vi "Continuous B sweep.vi"(6 "Mode":T5, 7 "Rate (T/min)":dbl=0.0125 min=0.0 max=0.2, 8 "error in (no error)":errorcluster, 9 "Simulate/Run":enum16{"simulate mode", "run mode"}(ring), 10 "Min (start)":dbl=1.0 min=-8.0 max=8.0, 11 "Max (end)":dbl=-1.0 min=-8.0 max=8.0) -> (0 "error out":errorcluster)   [LabVIEW 2019, in "Sweep Control.lvclass"]
uses:
  Sweep Control.lvclass
  Typedefs/Enum - Experiments.ctl
  Typedefs/Continuous B Sweep JSON--Cluster.ctl
  <userlib>/LevyLab/Instrument Framework/Instrument Types/Cryostat/Instrument.Cryostat.lvclass
  <userlib>/LevyLab/Transport/Transport/Transport.lvclass
  <userlib>/LevyLab/Transport/Control Experiment/Control Experiment.lvclass
  <userlib>/LevyLab/Lockin-Multichannel/Instrument.Lockin/Instrument.Lockin.lvclass
  <userlib>/LevyLab/Transport/Control Experiment/Typedefs/Instrument Classes--cluster.ctl
  <userlib>/LevyLab/Transport/Control Experiment/Typedefs/Wiring Description--cluster.ctl
  <userlib>/LevyLab/Transport/Control Experiment/Typedefs/Instrument--enum.ctl
  <userlib>/LevyLab/Transport/Control Experiment/Typedefs/Experiment Description--cluster.ctl
  <userlib>/LevyLab/Instrument Framework/Instrument Types/VSource/Instrument.VSource.lvclass
  <userlib>/LevyLab/Instrument Framework/Instrument Types/VNA/Instrument.VNA.lvclass
  <userlib>/LevyLab/Instrument Framework/Instrument Types/Strain/Instrument.Strain.lvclass
  <userlib>/LevyLab/Instrument Framework/Instrument Types/CBridge/Instrument.CBridge.lvclass
  <userlib>/LevyLab/Lockin-Multichannel/Instrument.DAQ/Typedefs/Sweep.Pattern--Enum.ctl
  <userlib>/LevyLab/Lockin-Multichannel/Instrument.DAQ/Instrument.DAQ.lvclass
  <userlib>/LevyLab/Lockin-Multichannel/Instrument.DAQ/Typedefs/Sweep.Channel--Cluster.ctl
  <userlib>/LevyLab/Instrument Framework/Instrument Types/Delay Line/Instrument.DelayLine.lvclass
  <userlib>/LevyLab/Transport/Control Experiment/Typedefs/Instrument Types--combo.ctl
  <userlib>/LevyLab/Lockin-Multichannel/Instrument.DAQ/Typedefs/REF.Channel--Cluster.ctl
  <userlib>/LevyLab/Lockin-Multichannel/Instrument.DAQ/Typedefs/REF.Channel--Cluster--Array.ctl
  <userlib>/LevyLab/Lockin-Multichannel/Instrument.DAQ/Typedefs/AO.Channel.Function--Enum.ctl
  <userlib>/LevyLab/Lockin-Multichannel/Instrument.DAQ/Typedefs/AO.Channel--Cluster.ctl
  <userlib>/LevyLab/Lockin-Multichannel/Instrument.DAQ/Typedefs/AO.Channel--Cluster--Array.ctl
  65c9b652-50f2-4ab4-8260-00ea008a43cc.vi
  <userlib>/LevyLab/Transport/Control Experiment/Typedefs/Instruments--cluster.ctl
  <userlib>/LevyLab/Krohn Hite 7008/SMOs/Inst.Krohn-Hite-7008/Inst.Krohn-Hite-7008.lvclass
  <userlib>/LevyLab/Krohn Hite 7008/SMOs/KH7008/typedefs/Filter--Enum.ctl
  <userlib>/LevyLab/Krohn Hite 7008/SMOs/KH7008/KH7008.lvlib
  <userlib>/LevyLab/Krohn Hite 7008/SMOs/KH7008/typedefs/couple--Enum.ctl
  <userlib>/LevyLab/Krohn Hite 7008/SMOs/KH7008/typedefs/shunt--enum.ctl
  <userlib>/LevyLab/Krohn Hite 7008/SMOs/KH7008/typedefs/Input--Enum.ctl
  <userlib>/LevyLab/Krohn Hite 7008/SMOs/KH7008/typedefs/gain--enum.ctl
  <userlib>/LevyLab/Krohn Hite 7008/SMOs/KH7008/typedefs/channel--numeric.ctl
  <userlib>/LevyLab/Krohn Hite 7008/SMOs/KH7008/typedefs/channelProperties--Cluster.ctl
  <userlib>/LevyLab/Krohn Hite 7008/SMOs/KH7008/typedefs/allChannelProperties--Array.ctl
  <userlib>/LevyLab/Instrument Framework/Instrument Types/Cryostat/Typedefs/Magnet Mode--Enum.ctl
  <userlib>/LevyLab/Lockin-Multichannel/Instrument.DAQ/Typedefs/Sweep.Channel--Cluster--Array.ctl
  <userlib>/LevyLab/Transport/Transport/Typedefs/Lockin_Sweep JSON--Cluster.ctl
panel:
  in  "Lockin_sweep Configuration":T1[](array[typedef]) {"Sweep Tables"."Table" format="%#_3p"; "Sweep Tables"."Ch" min=1 max=16; "Sweep Channels"."Table" format="%#_1f"; "Sweep Channels"."Channel" min=1 max=128; "Sweep Channels"."Start" format="%#_6p"; "Sweep Channels"."End" format="%#_6p"}
  out "Setpoint (T)":dbl=1.0
  in  "Experiment Folder":string="49-LockinFieldSweep"
  in  "Experiment subVI":T6
  in  "Experiment Description":string="Lockin measurements at different X and Y gate values\n\n- lockin channel 17,18,19,20: leads 3,8,15,27 (x,y,-x,-y gates)\ngate combinations:\nx2,y2,x1,y1\n0,0,0,0\n17.5,0,-17.5,0\n-17.5,0,17.5,0\n0,17.5,0,-17.5\n0,-17.5,0,17.5\n17.5,0,17.5,0\n0,17.5,0,17.5\n\n-Vbg = lead 26: 0V\n-T: 20mK\n-B=1T to -1T @0.0125T/min and vice versa\n\n400nm periodicity hash\n\nLockin channel 2,1: leads 5,4 , current mode, SR: 5kOhm, Gain:1000x\nLockin channel 2: lead 5: Vac:1mV, Vdc:0V, freq: 13Hz\nLockin channel 3,4: leads 6,7 , voltage mode SR: open, Gain:1000x\n\nsolid rectangle\n    \nLockin channel 5,8: leads 9,13 , current mode, SR: 5kOhm, Gain:1000x\nLockin channel 5: lead 9: Vac:1mV, Vdc:0V, freq: 13Hz\nLockin channel 6,7: leads 11,12 , voltage mode SR: open, Gain:1000x\n\n\n200nm periodicity hash\n\nLockin channel 12,11: leads 21,20 , current mode, SR: 5kOhm, Gain:1000x\nLockin channel 12: lead 21: Vac:1mV, Vdc:0V, freq: 13Hz\nLockin channel 9,10: leads 16,17 , voltage mode SR: open, Gain:1000x\n\nAdditional lockin settings:\nLine filter on\nDecimation Factor: 10\nFs: 65000\n#s: 5000"
  out "time (minutes)":dbl=40.0
  out "ETA":timestamp=timestamp(3698546516.7356124 s since 1904-01-01) caption="Timestamp" format="%<%m/%d/%Y %I:%M:%S %p>T"
  out "time (hours)":dbl=2.0
  out "Step #":i32=1
  in  "Function":enum16{"Ramp", "Triangle", "Sine"}(ring)
  in  "Phase":dbl
  in  "Cycles (1,2,...)":i32=1 min=1 step=1
  in  "step size":dbl=2.0 format="%.4f"
  out "B Field Graph":cluster{i32[], dbl[]}[](graph)=[{[0, 1], [-1.0, 1.0]}, {[1], [1.0]}]
  in  "stop":bool
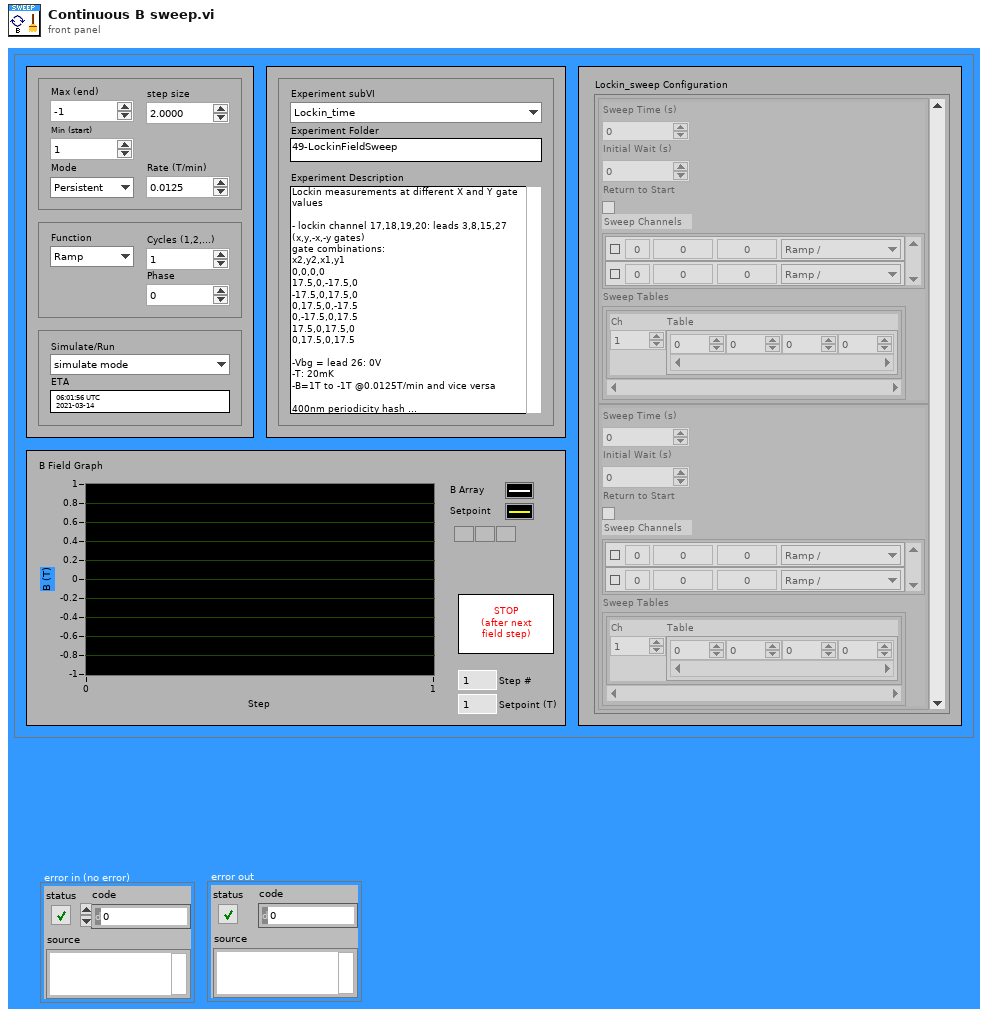
[diagram p1: front panel]
types:
  T1 = typedef "Transport.lvclass/Lockin_Sweep JSON--Cluster.ctl" = cluster{"Sweep Time (s)":dbl, "Initial Wait (s)":dbl, "Return to Start":bool, "Sweep Channels":T2, "Sweep Tables":cluster{"Ch":i32, "Table":dbl[]}[]}
  T2 = typedef "Instrument.DAQ.lvclass/Sweep.Channel--Cluster--Array.ctl" = T3[]
  T3 = typedef "Instrument.DAQ.lvclass/Sweep.Channel--Cluster.ctl" = cluster{"Enable?":bool, "Channel":u16, "Start":dbl, "End":dbl, "Pattern":T4, "Table":dbl[]}
  T4 = typedef "Instrument.DAQ.lvclass/Sweep.Pattern--Enum.ctl" = enum16{"Ramp /", "Ramp /\\", "Smooth Ramp _/", "Smooth Ramp _/\\_", "Table"}
  T5 = typedef "Instrument.Cryostat.lvclass/Magnet Mode--Enum.ctl" = enum16{"Persistent", "Driven"}
  T6 = typedef "Sweep Control.lvclass/Enum - Experiments.ctl" = enum16{"Lockin_time", "Lockin_sweep", "Lockin_DelayLine"}
  T7 = cluster{"Sweep Time (s)":dbl, "Initial Wait (s)":dbl, "Return to Start":bool, "Channels":T3[]}
  T8 = enum32{"Invalid", "Standard", "Closed", "Hidden", "Minimized", "Maximized"}
  T9 = enum32{"invalid app kind", "Development System", "Run Time System", "Student Edition", "Embedded LabVIEW", "Evaluation", "Custom"}
  T10 = typedef "Sweep Control.lvclass/Continuous B Sweep JSON--Cluster.ctl" = cluster{"Continuous B Sweep":cluster{"Experiment":T6, "B field values":dbl[]}, "Experiment Description":T11, "Wiring Configuration":T15, "Lockin":cluster{"AOconfig":T16, "REFconfig":T19}, "Krohn Hite":cluster{"Channel Setting":T21}}
  T11 = typedef "Control Experiment.lvclass/Experiment Description--cluster.ctl" = cluster{"User":string, "Device":string, "Device Path":path, "Device Description":string, "Experiment Path":path, "Experiment Description":string, "Instrument":T12, "Instruments":T13[], "Sweep":cluster{"key":string, "value":variant}[]}
  T12 = typedef "Control Experiment.lvclass/Instrument--enum.ctl" = enum16{"----- AFM/EBL -----", "AGILENT", "CYPHER", "Gemini2", "JEOL", "MFP3D", "----- Cryostat -----", "CF900", "DR200", "MNK", "PPMS (simulated)", "PPMS 1", "PPMS 2", "PPMS 3", "----- Optics -----", "THz 1 (Element 2/Montana)", "THz 2 (Tsunami/Janis)"}
  T13 = typedef "Control Experiment.lvclass/Instruments--cluster.ctl" = cluster{"class path":path, "Address":string, "Type":T14}
  T14 = typedef "Control Experiment.lvclass/Instrument Types--combo.ctl" = string
  T15 = typedef "Control Experiment.lvclass/Wiring Description--cluster.ctl" = cluster{"Lockin Ch":i32[], "KH":cluster{"Electrodes":string[], "Labels":string[]}, "not KH":cluster{"Electrodes":string[], "Labels":string[]}}
  T16 = typedef "Instrument.DAQ.lvclass/AO.Channel--Cluster--Array.ctl" = T17[]
  T17 = typedef "Instrument.DAQ.lvclass/AO.Channel--Cluster.ctl" = cluster{"Enable?":bool, "Channel":i32, "Amplitude":dbl, "Offset":dbl, "Frequency":dbl, "Phase":dbl, "Function":T18, "Sweeping?":bool}
  T18 = typedef "Instrument.DAQ.lvclass/AO.Channel.Function--Enum.ctl" = enum16{"Sine", "Triangle", "Square"}
  T19 = typedef "Instrument.DAQ.lvclass/REF.Channel--Cluster--Array.ctl" = T20[]
  T20 = typedef "Instrument.DAQ.lvclass/REF.Channel--Cluster.ctl" = cluster{"Enable?":bool, "Channel":i32, "Frequency":dbl, "Phase":dbl, "TC":dbl, "Roll-Off":i32}
  T21 = typedef "KH7008.lvlib/allChannelProperties--Array.ctl" = T22[]
  T22 = typedef "KH7008.lvlib/channelProperties--Cluster.ctl" = cluster{"channel":T23, "gain":T24, "input":T25, "shunt":T26, "couple":T27, "filter":T28}
  T23 = typedef "KH7008.lvlib/channel--numeric.ctl" = u16
  T24 = typedef "KH7008.lvlib/gain--enum.ctl" = enum16{"1x", "10x", "100x", "1000x"}
  T25 = typedef "KH7008.lvlib/Input--Enum.ctl" = enum16{"OFF", "SE+", "SE-", "DIFF"}
  T26 = typedef "KH7008.lvlib/shunt--enum.ctl" = enum16{"Open", "50", "500", "5k", "50k", "10M"}
  T27 = typedef "KH7008.lvlib/couple--Enum.ctl" = enum16{"AC", "DC"}
  T28 = typedef "KH7008.lvlib/Filter--Enum.ctl" = enum16{"OFF", "ON"}
  T29 = typedef "Control Experiment.lvclass/Instrument Classes--cluster.ctl" = cluster{"KH7008":refnum<class "Inst.Krohn-Hite-7008.lvclass">, "Lockin":refnum<class "Instrument.Lockin.lvclass">, "Temperature":refnum<class "Instrument.Cryostat.lvclass">, "Magnet":refnum<class "Instrument.Cryostat.lvclass">, "Rotator":refnum<class "Instrument.Cryostat.lvclass">, "Level":refnum<class "Instrument.Cryostat.lvclass">, "Capacitance Bridge":refnum<class "Instrument.CBridge.lvclass">, "Delay Line":refnum<class "Instrument.DelayLine.lvclass">, "Strain Cell":refnum<class "Instrument.Strain.lvclass">, "VNA":refnum<class "Instrument.VNA.lvclass">, "Voltage Source":refnum<class "Instrument.VSource.lvclass">}
  T30 = cluster{"Core":cluster{"Current VI Reference":refnum<vi>, "Close Panel on Exit?":bool}, "SweepControl":refnum<class "Sweep Control.lvclass">, "ContinuousB_JSON":T10, "B field values":dbl[], "Sweep rate (T/min)":dbl, "Transport":refnum<class "Transport.lvclass">, "Instruments":T29, "Notifier":refnum<notifier>}
  T31 = cluster{"Current VI Reference":refnum<vi>, "Close Panel on Exit?":bool}
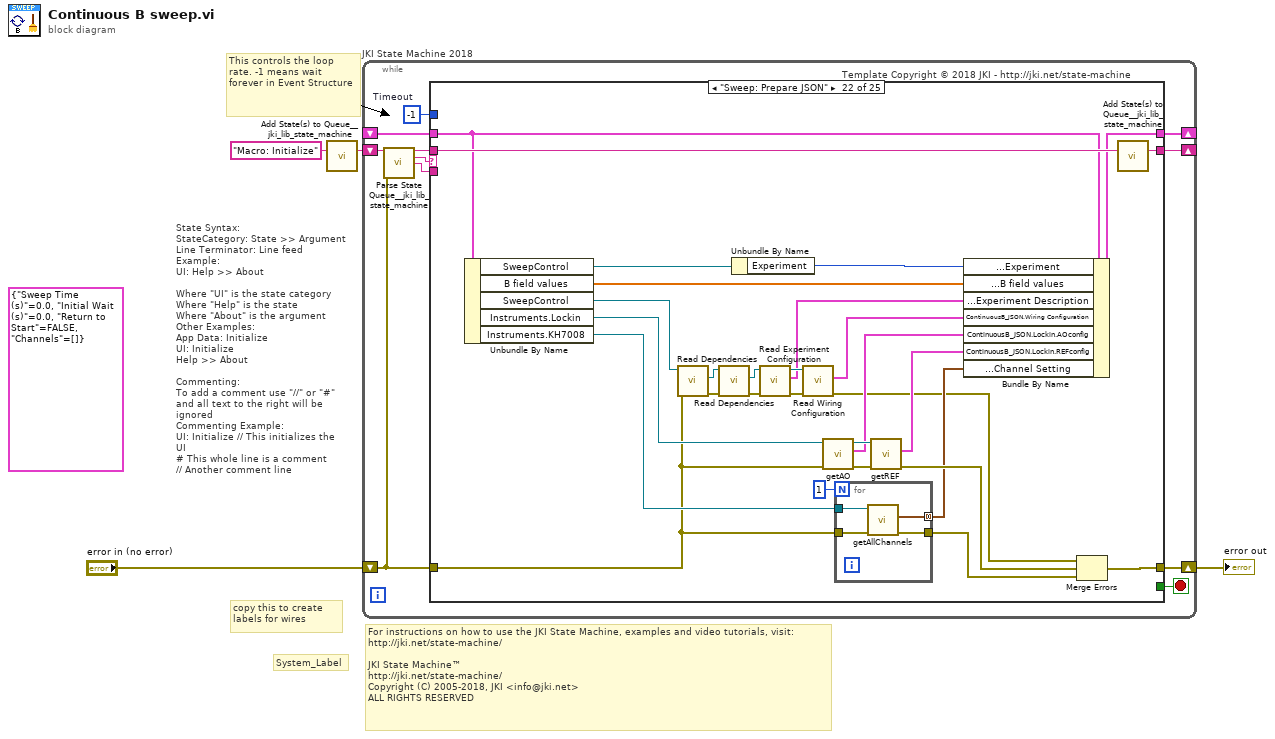
[diagram p0: block diagram]
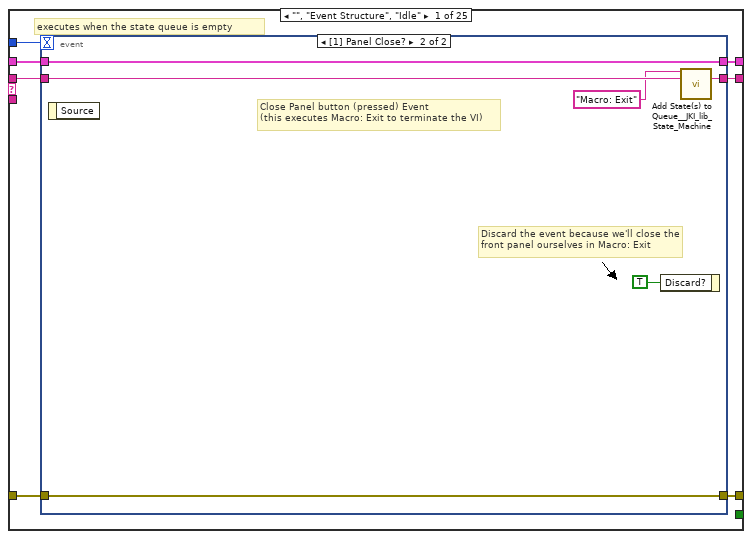
[diagram p2: hidden frame]
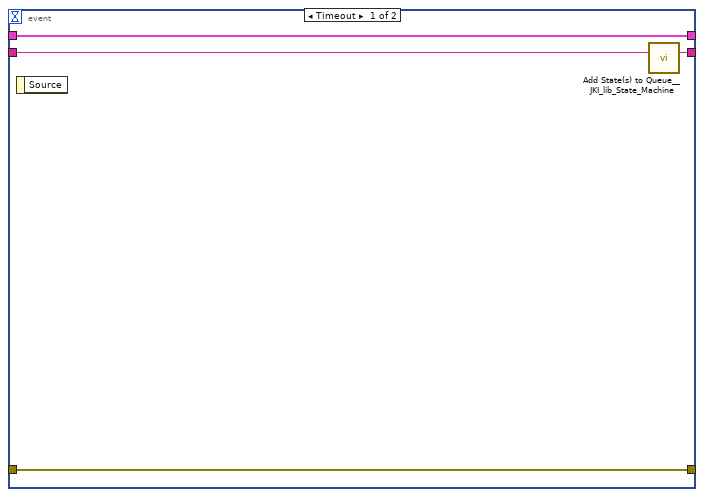
[diagram p3: hidden frame]
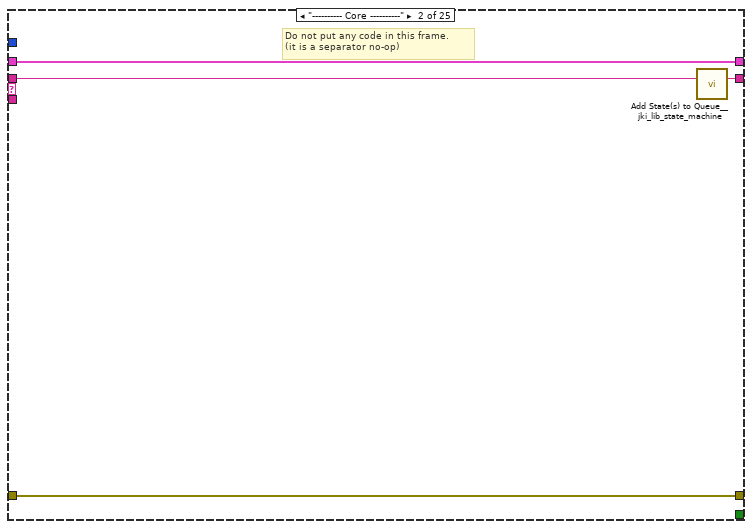
[diagram p4: hidden frame]
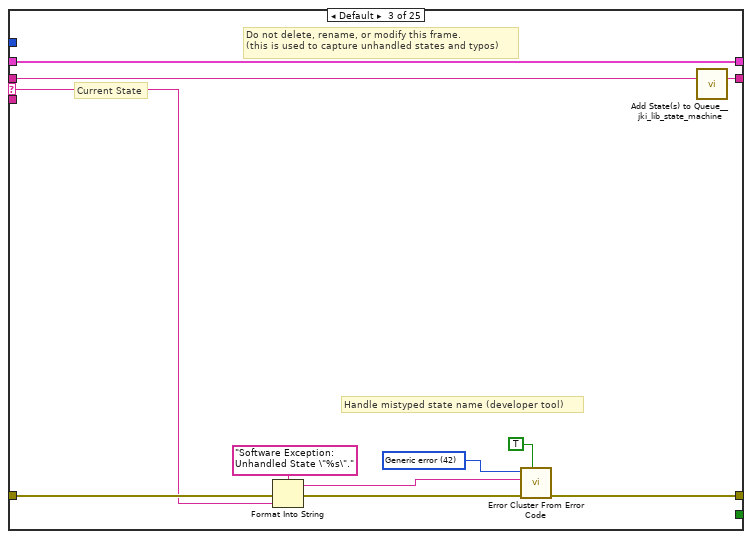
[diagram p5: hidden frame]
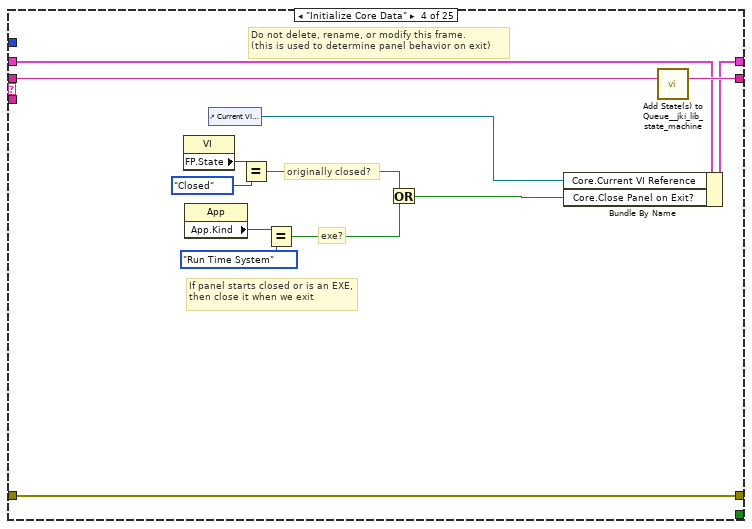
[diagram p6: hidden frame]
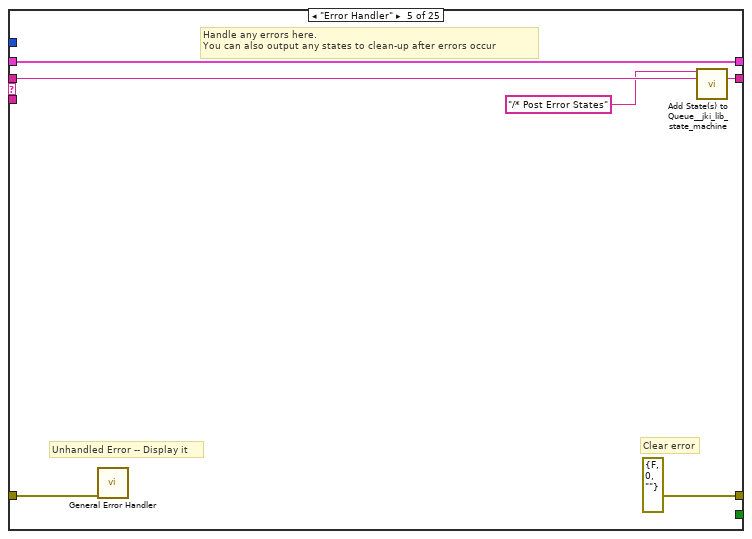
[diagram p7: hidden frame]
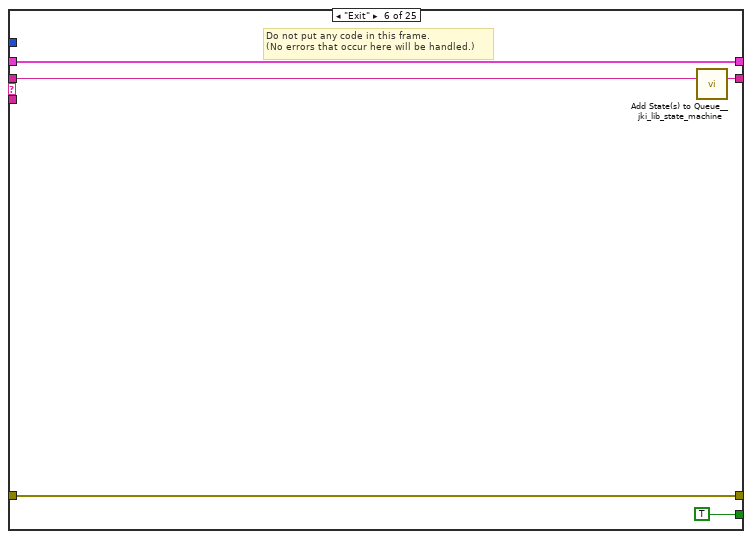
[diagram p8: hidden frame]
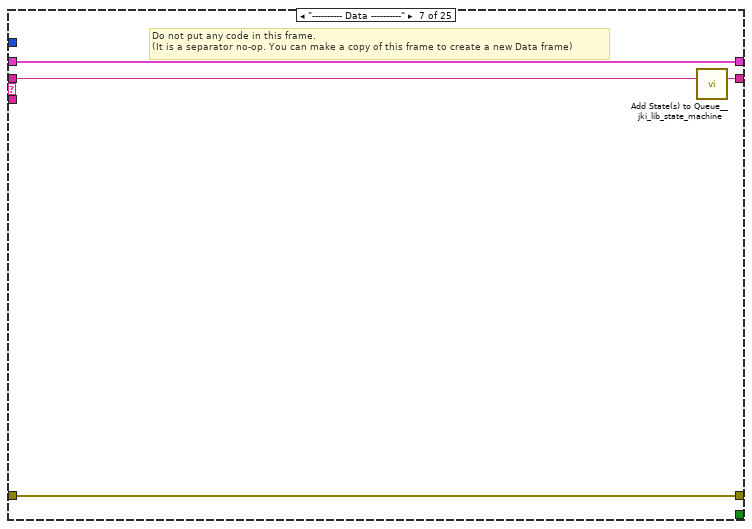
[diagram p9: hidden frame]
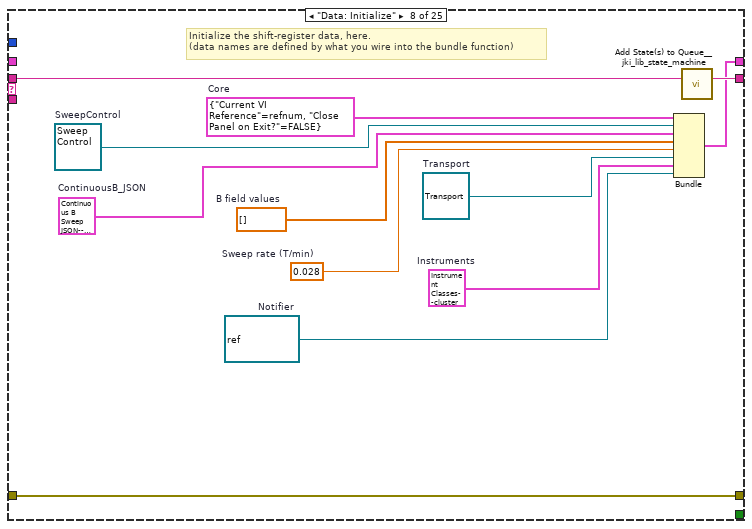
[diagram p10: hidden frame]
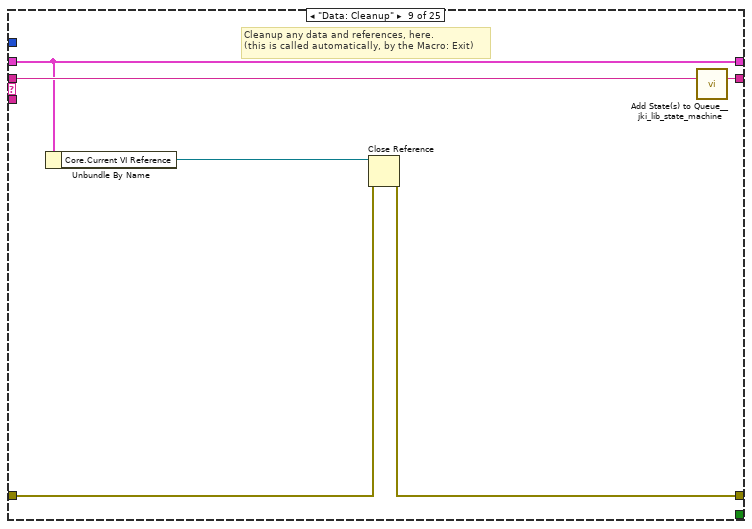
[diagram p11: hidden frame]
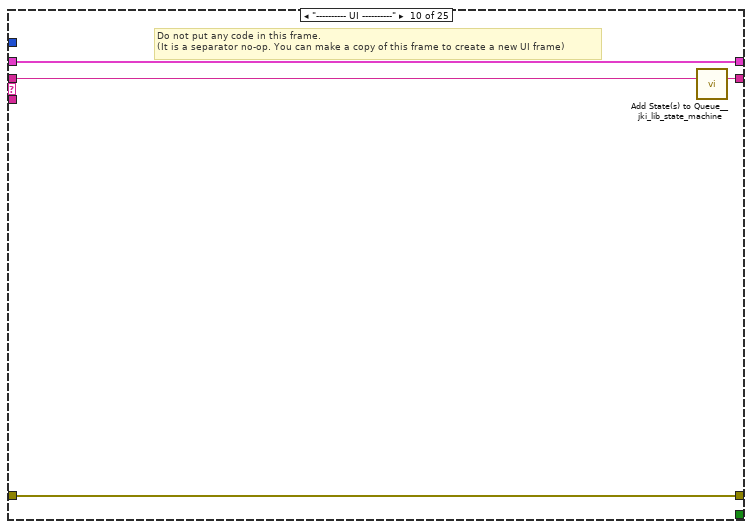
[diagram p12: hidden frame]
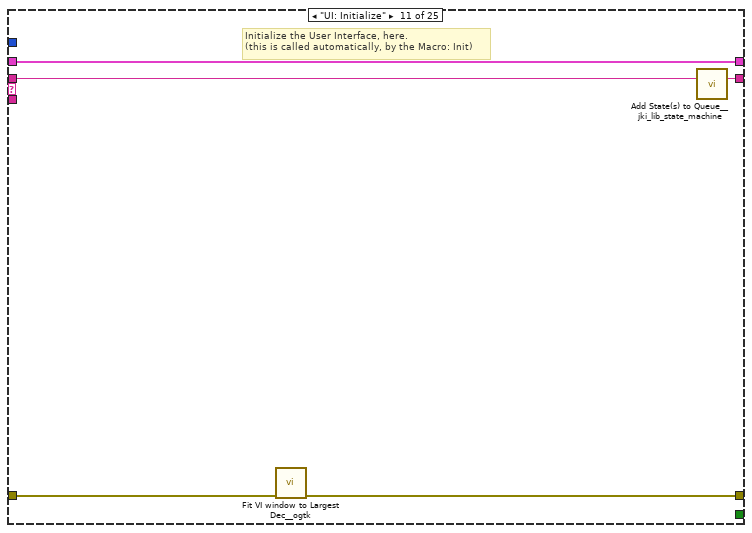
[diagram p13: hidden frame]
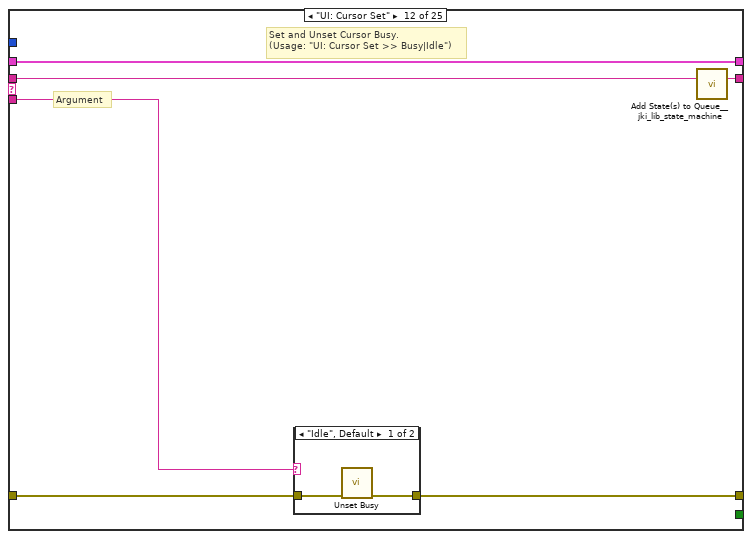
[diagram p14: hidden frame]
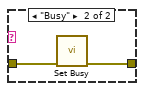
[diagram p15: hidden frame]
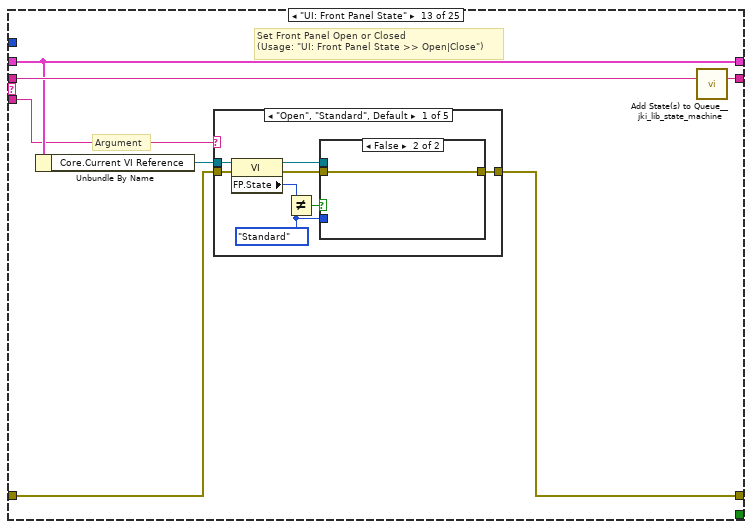
[diagram p16: hidden frame]
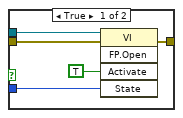
[diagram p17: hidden frame]
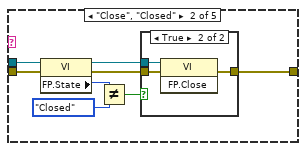
[diagram p18: hidden frame]
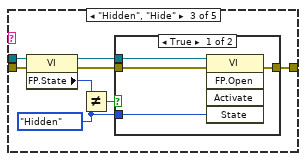
[diagram p20: hidden frame]
diagram:
  (unwired) T7 {"Sweep Time (s)"=0.0, "Initial Wait (s)"=0.0, "Return to Start"=FALSE, "Channels"=[]} ("Sweep")
  # "For instructions on how to use the JKI State Machine, examples and video tutorials, visit:\nhttp://jki.net/state-machine/\n\nJKI State Machine™\nhttp://jki.net/state-machine/\nCopyright (C) 2005-2018, JKI <info@jki.net>\nALL RIGHTS RESERVED"
  # "State Syntax:\nStateCategory: State >> Argument\nLine Terminator: Line feed\nExample:\nUI: Help >> About\n\nWhere \"UI\" is the state category\nWhere \"Help\" is the state\nWhere \"About\" is the argument\nOther Examples:\nApp Data: Initialize\nUI: Initialize\nHelp >> About\n\nCommenting:\nTo add a comment use \"//\" or \"#\" and all text to the right will be ignored\nCommenting Example:\nUI: Initialize // This initializes the UI\n# This whole line is a comment\n// Another comment line"
  # "copy this to create labels for wires"
  # "This controls the loop rate. -1 means wait forever in Event Structure"
  # "System_Label"
  n1 = call <vilib>:"Add State(s) to Queue__jki_lib_state_machine.vi"("State(s) in (\"\")"="Macro: Initialize") -> ("States Out"=w4:string)  [unwired: 14 in]
  n2 = while "JKI State Machine 2018" {
    shift-right: [w8] -> _
    shift-left: _ -> [w7]
    shift-right: [w11] -> w1
    shift-left: "error in (no error)" -> [w5]
    shift-right: [w10] -> _
    shift-left: w4 -> [w12]
    stop <- w9 stop-if-true
    w6 = -1  # Timeout
    # "Template Copyright © 2018 JKI - http://jki.net/state-machine"
    n3 = call <vilib>:"Parse State Queue__jki_lib_state_machine.vi"("State Queue"=w12, "Error In (no error)"=w5) -> ("Remaining States"=w14:string, "Current State"=w15:string, "Arguments"=w13:string)  [unwired: 11 in]
    n4 = case shown="\"Sweep: Prepare JSON\"" w15 {
      selector: w15 -> [_ _ w37 _ _ _ _ _ _ _ _ _ _ _ _ _ _ _ _ _ _ _ _ _ _]
      tunnel: w14 -> [w22 w36 w41 w60 w66 w71 w75 w87 w93 w97 w102 w108 w119 w188 w193 w199 w211 w215 w234 w260 w274 w303 w331 w348 w387]
      tunnel: w13 -> [_ _ _ _ _ _ _ _ _ _ _ w103 w113 _ _ _ _ _ _ _ _ _ _ _ _]
      tunnel: w7 -> [w20 w33 w39 w53 w63 w69 w72 _ w88 w94 w100 w106 w115 w185 w190 w196 w208 w212 w224 w246 w270 w295 w329 w335 w372]
      tunnel: [w19 w34 w43 w57 errorcluster {"status"=FALSE, "code"=0, "source"=""} ("error out") w68 w73 w84 w89 w95 w98 w104 w116 w186 w191 w197 w209 w213 w222 w237 w268 w288 w313 w346 w377] -> w11
      tunnel: w5 -> [w18 w34 w42 w57 w62 w68 w73 w84 w90 w95 w99 w105 w117 w186 w191 w197 w209 w213 w222 w250 w269 w276 w318 w346 w380]
      tunnel: [w21 w35 w40 w59 w65 w70 w74 w86 w92 w96 w101 w107 w118 w187 w192 w198 w210 w214 w233 w259 w273 w302 w330 w347 w386] -> w10
      tunnel: [_ _ _ _ _ TRUE _ _ _ _ _ _ _ _ _ _ _ _ _ _ _ _ _ _ _] -> w9
      tunnel: [w17 w33 w39 w58 w63 w69 w72 w85 w88 w94 w100 w106 w115 w185 w190 w196 w208 w212 w232 w245 w271 w294 w328 w335 w371] -> w8
      tunnel: w6 -> [w16 _ _ _ _ _ _ _ _ _ _ _ _ _ _ _ _ _ _ _ _ _ _ _ _]
      frame "", "Event Structure", "Idle" {
        # "executes when the state queue is empty"
        n5 = event shown="[1] Panel Close?" {
          selector: _ -> [_ _]
          dyn-events: _ -> [_ _]
          timeout: w16 -> [_ _]
          tunnel: w22 -> [w26 w32]
          tunnel: [w25 w31] -> w21
          tunnel: w20 -> [w23 w29]
          tunnel: [w24 w30] -> w19
          tunnel: w18 -> [w24 w30]
          tunnel: [w23 w29] -> w17
          event Timeout {
            n6 = event-data() -> ()  [unwired: 1 in, 1 out]
            n7 = call <vilib>:"Add State(s) to Queue__JKI_lib_State_Machine.vi"("State(s) in (\"\")"=w26) -> ("States Out"=w25:string)  [unwired: 14 in]
          }
          event Panel Close? {
            # "Discard the event because we'll close the front panel ourselves in Macro: Exit"
            # "Close Panel button (pressed) Event\n(this executes Macro: Exit to terminate the VI)"
            n8 = event-data() -> ()  [unwired: 1 in, 1 out]
            n9 = event-data("Discard?"=TRUE) -> ()  [unwired: 1 in, 1 out]
            n10 = call <vilib>:"Add State(s) to Queue__JKI_lib_State_Machine.vi"("State(s) in Front (\"\")"="Macro: Exit", "State(s) in (\"\")"=w32) -> ("States Out"=w31:string)  [unwired: 13 in]
          }
        }
      }
      frame "---------- Core ----------" {
        # "Do not put any code in this frame.\n(it is a separator no-op)"
        n11 = call <vilib>:"Add State(s) to Queue__jki_lib_state_machine.vi"("State(s) in (\"\")"=w36) -> ("States Out"=w35:string)  [unwired: 14 in]
      }
      frame Default {
        w46 = 42 items=["No error", "Argument error", "Memory is full", "Out of zone", "End of file", "File already open", "Generic file I/O error", "File not found", "File permission error", "Disk is full", "Duplicate path", "Too many files open", "System feature not enabled", "Resource file not found", "Cannot add resource", "Resource not found", "Image not found", "Image memory error", "Pen does not exist", "Config type invalid", "Config token not found", "Config parse error", "Config memory error", "Bad external code format", "Bad external code offset", "External code not present", "Null window", "Destroy window error", "Null menu", "Print aborted", "Bad print record", "Print driver error", "Windows error during printing", "Memory error during printing", "Print dialog error", "Generic print error", "Invalid device refnum", "Device not found", "Device parameter error", "Device unit error", "Cannot open device", "Device call aborted", "Generic error", "Cancelled by user", "Object ID too low", "Object ID too high", "Object not in heap", "Unknown heap", "Unknown object (invalid DefProc)", "Unknown object (DefProc not in table)", "Message out of range", "Invalid (null) method", "Unknown message", "Manager call not supported", "Bad address", "Network operation in progress", "Network operation timed out", "Connection is busy", "Network attribute not supported", "Network error", "Address in use", "System out of memory", "Connection aborted", "Connection refused", "Not connected", "Already connected", "Connection closed", "Initialization error (interapplication manager)", "Bad occurrence", "Wait on unbound occurrence handler", "Occurrence queue overflow", "Datalog type conflict", "Unused", "Unrecognized type (interapplication manager)", "Memory corrupt", "Failed to make temporary DLL", "Old CIN version", "Drag socket not found", "Failed to load drop-object", "Failed to register OLE object", "Failed to release OLE object", "Format specifier type mismatch", "Unknown format specifier", "Too few format specifiers", "Too many format specifiers", "Scan failed", "Newer CIN version", "Error converting to variant", "Runtime menu error", "Password tampered", "Variant attribute not found", "Incompatible variant data type", "Event data is not available", "Event Store is not present", "Occurrence is not found", "Event Queue is not created", "Event info is not available", "Refnum passed is NULL", "Error retrieving Class GUID", "Error retrieving CoClass GUID", "Error retrieving TypeLib GUID.", "Bad built application magic bytes.", "Specific driver is different from the specific driver associated with the Logical Name.", "There is no session opened to the class driver.", "Max Error", "MAX - Error with config objects", "MAX - Error loading configuration", "MAX - Group not supported"]
        # "Current State"
        # "Do not delete, rename, or modify this frame.\n(this is used to capture unhandled states and typos)"
        # "Handle mistyped state name (developer tool)"
        n12 = Format Into String(format string="Software Exception: Unhandled State \"%s\"." ("message"), error in=w42, w37) -> (resulting string=w45:string, error out=w44:errorcluster)  [unwired: 1 in]
        n13 = call <vilib>:"Error Cluster From Error Code.vi"("show call chain? (False)"=TRUE, "error in (no error)"=w44, "error message (\"\")"=w45, "error code (0)"=w46) -> ("error out"=w43:errorcluster)  [unwired: 5 in]
        n14 = call <vilib>:"Add State(s) to Queue__jki_lib_state_machine.vi"("State(s) in (\"\")"=w41) -> ("States Out"=w40:string)  [unwired: 14 in]
      }
      frame "Initialize Core Data" {
        # "Do not delete, rename, or modify this frame.\n(this is used to determine panel behavior on exit)"
        # "originally closed?"
        # "exe?"
        # "If panel starts closed or is an EXE, then close it when we exit"
        n15 = property class="VI"() -> ("FP.State"=w50:T8)  [unwired: 2 in, 2 out]
        n16 = property class="App"() -> ("App.Kind"=w56:T9)  [unwired: 2 in, 2 out]
        n17 = control-ref of="Current VI Reference"() -> (w51:refnum<vi>)
        n18 = Equal?(x=w50, y=T8."Closed" ("Front Panel Window:State")) -> (x = y?=w48:bool)
        n19 = Equal?(x=w56, y=T9."Run Time System" ("Application:Kind")) -> (x = y?=w54:bool)
        n20 = Or(x=w48, y=w54) -> (x .or. y?=w52:bool)
        n21 = Bundle By Name(cluster=w53, "Core.Current VI Reference"=w51, "Core.Close Panel on Exit?"=w52) -> (w58:T30)
        n22 = call <vilib>:"Add State(s) to Queue__jki_lib_state_machine.vi"("State(s) in (\"\")"=w60) -> ("States Out"=w59:string)  [unwired: 14 in]
      }
      frame "Error Handler" {
        # "Unhandled Error -- Display it"
        # "Handle any errors here.\nYou can also output any states to clean-up after errors occur"
        # "Clear error"
        n23 = call <vilib>:"General Error Handler.vi"("error in (no error)"=w62) -> ()  [unwired: 10 in, 5 out]
        n24 = call <vilib>:"Add State(s) to Queue__jki_lib_state_machine.vi"("State(s) in Front (\"\")"="/* Post Error States", "State(s) in (\"\")"=w66) -> ("States Out"=w65:string)  [unwired: 13 in]
      }
      frame "Exit" {
        # "Do not put any code in this frame.\n(No errors that occur here will be handled.)"
        n25 = call <vilib>:"Add State(s) to Queue__jki_lib_state_machine.vi"("State(s) in (\"\")"=w71) -> ("States Out"=w70:string)  [unwired: 14 in]
      }
      frame "---------- Data ----------" {
        # "Do not put any code in this frame.\n(It is a separator no-op. You can make a copy of this frame to create a new Data frame)"
        n26 = call <vilib>:"Add State(s) to Queue__jki_lib_state_machine.vi"("State(s) in (\"\")"=w75) -> ("States Out"=w74:string)  [unwired: 14 in]
      }
      frame "Data: Initialize" {
        w76 = T10 {"Continuous B Sweep"={"Experiment"=enum."Lockin_DelayLine", "B field values"=[]}, "Experiment Description"={"User"="", "Device"="", "Device Path"=path "", "Device Description"="", "Experiment Path"=path "", "Experiment Description"="", "Instrument"=enum."PPMS 1", "Instruments"=[], "Sweep"=[]}, "Wiring Configuration"={"Lockin Ch"=[], "KH"={"Electrodes"=[], "Labels"=[]}, "not KH"={"Electrodes"=[], "Labels"=[]}}, "Lockin"={"AOconfig"=[], "REFconfig"=[]}, "Krohn Hite"={"Channel Setting"=[]}}  # ContinuousB_JSON
        w77 = T29 {"KH7008"=refnum, "Lockin"=refnum, "Temperature"=refnum, "Magnet"=refnum, "Rotator"=refnum, "Level"=refnum, "Capacitance Bridge"=refnum, "Delay Line"=refnum, "Strain Cell"=refnum, "VNA"=refnum, "Voltage Source"=refnum}  # Instruments
        w79 = refnum<class "Transport.lvclass"> refnum  # Transport
        w80 = refnum<class "Sweep Control.lvclass"> refnum  # SweepControl
        w78 = refnum<notifier> refnum  # Notifier
        w81 = 0.028  # Sweep rate (T/min)
        w82 = dbl[] []  # B field values
        w83 = T31 {"Current VI Reference"=refnum, "Close Panel on Exit?"=FALSE}  # Core
        # "Initialize the shift-register data, here.\n(data names are defined by what you wire into the bundle function)"
        n27 = Bundle("Core"=w83, "SweepControl"=w80, "ContinuousB_JSON"=w76, "B field values"=w82, "Sweep rate (T/min)"=w81, "Transport"=w79, "Instruments"=w77, "Notifier"=w78) -> (w85:T30)  [unwired: 1 in]
        n28 = call <vilib>:"Add State(s) to Queue__jki_lib_state_machine.vi"("State(s) in (\"\")"=w87) -> ("States Out"=w86:string)  [unwired: 14 in]
      }
      frame "Data: Cleanup" {
        # "Cleanup any data and references, here.\n(this is called automatically, by the Macro: Exit)"
        n29 = Unbundle By Name(w88) -> ("Core.Current VI Reference"=w91:refnum<vi>)
        n30 = Close Reference(reference=w91, error in (no error)=w90) -> (error out=w89:errorcluster)
        n31 = call <vilib>:"Add State(s) to Queue__jki_lib_state_machine.vi"("State(s) in (\"\")"=w93) -> ("States Out"=w92:string)  [unwired: 14 in]
      }
      frame "---------- UI ----------" {
        # "Do not put any code in this frame.\n(It is a separator no-op. You can make a copy of this frame to create a new UI frame)"
        n32 = call <vilib>:"Add State(s) to Queue__jki_lib_state_machine.vi"("State(s) in (\"\")"=w97) -> ("States Out"=w96:string)  [unwired: 14 in]
      }
      frame "UI: Initialize" {
        # "Initialize the User Interface, here.\n(this is called automatically, by the Macro: Init)"
        n33 = call <userlib>:"Fit VI window to Largest Dec__ogtk.vi"("error in (no error)"=w99) -> ("error out"=w98:errorcluster)  [unwired: 5 in, 1 out]
        n34 = call <vilib>:"Add State(s) to Queue__jki_lib_state_machine.vi"("State(s) in (\"\")"=w102) -> ("States Out"=w101:string)  [unwired: 14 in]
      }
      frame "UI: Cursor Set" {
        # "Argument"
        # "Set and Unset Cursor Busy.\n(Usage: \"UI: Cursor Set >> Busy|Idle\")"
        n35 = case shown="\"Idle\", Default" w103 {
          tunnel: w105 -> [w110 w112]
          tunnel: [w109 w111] -> w104
          frame "Idle", Default {
            n36 = call <vilib>:"Unset Busy.vi"("error in (no error)"=w110) -> ("error out"=w109:errorcluster)  [unwired: 10 in]
          }
          frame "Busy" {
            n37 = call <vilib>:"Set Busy.vi"("error in (no error)"=w112) -> ("error out"=w111:errorcluster)  [unwired: 9 in, 1 out]
          }
        }
        n38 = call <vilib>:"Add State(s) to Queue__jki_lib_state_machine.vi"("State(s) in (\"\")"=w108) -> ("States Out"=w107:string)  [unwired: 14 in]
      }
      frame "UI: Front Panel State" {
        # "Argument"
        # "Set Front Panel Open or Closed\n(Usage: \"UI: Front Panel State >> Open|Close\")"
        n39 = Unbundle By Name(w115) -> ("Core.Current VI Reference"=w114:refnum<vi>)
        n40 = case shown="\"Open\", \"Standard\", Default" w113 {
          tunnel: w117 -> [w125 w140 w151 w164 w177]
          tunnel: [w127 w141 w153 w166 w179] -> w116
          tunnel: w114 -> [w126 w138 w152 w165 w178]
          frame "Open", "Standard", Default {
            w120 = T8."Standard" ("State")
            n41 = property class="VI"(reference=w126, error in=w125) -> (reference out=w123:refnum<vi>, error out=w124:errorcluster, "FP.State"=w122:T8)
            n42 = Not Equal?(x=w122, y=w120) -> (x != y?=w121:bool)
            n43 = case shown="False" w121 {
              tunnel: [w131 w133] -> w127
              tunnel: w124 -> [w130 w133]
              tunnel: w123 -> [w129 _]
              tunnel: w120 -> [w128 _]
              frame True {
                n44 = invoke class="VI" method="FP.Open"(reference=w129, error in=w130, "Activate"=TRUE, "State"=w128) -> (error out=w131:errorcluster)  [unwired: 1 in, 4 out]
              }
              frame False {
              }
            }
          }
          frame "Close", "Closed" {
            n45 = property class="VI"(reference=w138, error in=w140) -> (reference out=w137:refnum<vi>, error out=w139:errorcluster, "FP.State"=w135:T8)
            n46 = Not Equal?(x=w135, y=T8."Closed" ("Front Panel Window:State")) -> (x != y?=w134:bool)
            n47 = case shown="True" w134 {
              tunnel: [w142 w145] -> w141
              tunnel: w139 -> [w142 w144]
              tunnel: w137 -> [_ w143]
              frame False {
              }
              frame True {
                n48 = invoke class="VI" method="FP.Close"(reference=w143, error in=w144) -> (error out=w145:errorcluster)  [unwired: 1 in, 2 out]
              }
            }
          }
          frame "Hidden", "Hide" {
            w146 = T8."Hidden" ("State")
            n49 = property class="VI"(reference=w152, error in=w151) -> (reference out=w149:refnum<vi>, error out=w150:errorcluster, "FP.State"=w148:T8)
            n50 = Not Equal?(x=w148, y=w146) -> (x != y?=w147:bool)
            n51 = case shown="True" w147 {
              tunnel: [w157 w158] -> w153
              tunnel: w150 -> [w156 w158]
              tunnel: w149 -> [w155 _]
              tunnel: w146 -> [w154 _]
              frame True {
                n52 = invoke class="VI" method="FP.Open"(reference=w155, error in=w156, "State"=w154) -> (error out=w157:errorcluster)  [unwired: 2 in, 4 out]
              }
              frame False {
              }
            }
          }
          frame "Minimize", "Minimized" {
            w159 = T8."Minimized" ("State")
            n53 = property class="VI"(reference=w165, error in=w164) -> (reference out=w162:refnum<vi>, error out=w163:errorcluster, "FP.State"=w161:T8)
            n54 = Not Equal?(x=w161, y=w159) -> (x != y?=w160:bool)
            n55 = case shown="True" w160 {
              tunnel: [w170 w171] -> w166
              tunnel: w163 -> [w169 w171]
              tunnel: w162 -> [w168 _]
              tunnel: w159 -> [w167 _]
              frame True {
                n56 = invoke class="VI" method="FP.Open"(reference=w168, error in=w169, "State"=w167) -> (error out=w170:errorcluster)  [unwired: 2 in, 4 out]
              }
              frame False {
              }
            }
          }
          frame "Maximize", "Maximized" {
            w172 = T8."Maximized" ("State")
            n57 = property class="VI"(reference=w178, error in=w177) -> (reference out=w175:refnum<vi>, error out=w176:errorcluster, "FP.State"=w174:T8)
            n58 = Not Equal?(x=w174, y=w172) -> (x != y?=w173:bool)
            n59 = case shown="True" w173 {
              tunnel: [w183 w184] -> w179
              tunnel: w176 -> [w182 w184]
              tunnel: w175 -> [w181 _]
              tunnel: w172 -> [w180 _]
              frame True {
                n60 = invoke class="VI" method="FP.Open"(reference=w181, error in=w182, "State"=w180) -> (error out=w183:errorcluster)  [unwired: 2 in, 4 out]
              }
              frame False {
              }
            }
          }
        }
        n61 = call <vilib>:"Add State(s) to Queue__jki_lib_state_machine.vi"("State(s) in (\"\")"=w119) -> ("States Out"=w118:string)  [unwired: 14 in]
      }
      frame "---------- Macro ----------" {
        # "Do not put any code in this frame.\n(It is a separator no-op. You can make a copy of this frame to create a new Macro frame)"
        n62 = call <vilib>:"Add State(s) to Queue__jki_lib_state_machine.vi"("State(s) in (\"\")"=w188) -> ("States Out"=w187:string)  [unwired: 14 in]
      }
      frame "Macro: Initialize" {
        w189 = "Data: Initialize\nInitialize Core Data\nUI: Initialize\nUI: Front Panel State >> Open\nMacro: Sweep"  # Data: Initialize Initialize Core Data UI: Initialize UI: Front Panel State >> Open Macro: Sweep
        # "Initialization Macro\n(This is called once, when the VI starts)"
        n63 = call <vilib>:"Add State(s) to Queue__jki_lib_state_machine.vi"("State(s) in Front (\"\")"=w189, "State(s) in (\"\")"=w193) -> ("States Out"=w192:string)  [unwired: 13 in]
      }
      frame "Macro: Sweep" {
        # "Do not put any code in this frame.\n(It is a separator no-op. You can make a copy of this frame to create a new Macro frame)"
        n64 = case shown="\"simulate mode\", Default" "Simulate/Run" {
          tunnel: ["Sweep: Initialize\nSweep: Simulate Sweep\nMacro: Exit" "Sweep: Initialize\nSweep: Initialize Sweep Control\nSweep: Initialize Transport\nSweep: Prepare JSON\nSweep: Write JSON\nSweep: Sweep\nMacro: Exit"] -> w195
          frame "simulate mode", Default {
          }
          frame "run mode" {
          }
        }
        n65 = call <vilib>:"Add State(s) to Queue__jki_lib_state_machine.vi"("State(s) in Front (\"\")"=w195, "State(s) in (\"\")"=w199) -> ("States Out"=w198:string)  [unwired: 13 in]
      }
      frame "Macro: Exit" {
        # "Exit Macro\n(This is called once, when the VI exits)"
        n66 = Unbundle By Name(w208) -> ("Core.Close Panel on Exit?"=w207:bool)
        n67 = Select(t="UI: Front Panel State >> Close", s=w207, f="") -> (s? t:f=w204:string)
        n68 = call <vilib>:"Add State(s) to Queue__JKI_lib_State_Machine.vi"("State(s) in (\"\")"=w204, "State(s) at Back (\"\")"="Data: Cleanup\nExit") -> ("States Out"=w202:string)  [unwired: 13 in]
        n69 = call <vilib>:"Add State(s) to Queue__jki_lib_state_machine.vi"("State(s) in Front (\"\")"=w202, "State(s) in (\"\")"=w211) -> ("States Out"=w210:string)  [unwired: 13 in]
      }
      frame "---------- Sweep ----------" {
        # "Template Separator\n(You can make a copy of, or modify, this frame)"
        n70 = call <vilib>:"Add State(s) to Queue__jki_lib_state_machine.vi"("State(s) in (\"\")"=w215) -> ("States Out"=w214:string)  [unwired: 14 in]
      }
      frame "Sweep: Initialize" {
        # "Your code here.\n(You can make a copy of, or modify, this frame)"
        n71 = call <userlib>:"Max_Min_conversion.vi"("Min"="Min (start)", "Max"="Max (end)") -> ("offset"=w227:dbl, "Amplitude"=w226:dbl)  [unwired: 8 in]
        n72 = call <userlib>:"Ramp.vi"("phase"="Phase", "function (ramp)"="Function", "cycles (1,2,...)"="Cycles (1,2,...)", "step size"="step size", "offset"=w227, "amplitude"=w226) -> ("Waveform Graph"=w220:dbl[])  [unwired: 3 in, 2 out]
        n73 = for {
          tunnel: w220 -> [w235] mode=indexing
          tunnel: [w236] -> w219 mode=indexing
          tunnel: [w235] -> w218 mode=indexing
          i -> [w236]
        }
        n74 = Bundle(w219, w218) -> (w217:cluster{i32[], dbl[]})  [unwired: 1 in]
        n75 = Build Array(w217) -> (→"B Field Graph":cluster{i32[], dbl[]}[])
        n76 = Bundle By Name(cluster=w224, "B field values"=w220, "Sweep rate (T/min)"="Rate (T/min)") -> (w232:T30)
        n77 = call <vilib>:"Add State(s) to Queue__jki_lib_state_machine.vi"("State(s) in (\"\")"=w234) -> ("States Out"=w233:string)  [unwired: 14 in]
      }
      frame "Sweep: Initialize Sweep Control" {
        # "Template Separator\n(You can make a copy of, or modify, this frame)"
        n78 = Unbundle By Name(w246) -> ("SweepControl"=w251:refnum<class "Sweep Control.lvclass">)
        n79 = call <userlib>:"Control Experiment FGV.vi"("Function"=enum16{"read", "write"}."read", "error in (no error)"=w250) -> ("error out"=w247:errorcluster, "Control Experiment.lvclass out"=w256:refnum<class "Control Experiment.lvclass">)  [unwired: 8 in]
        n80 = Bundle By Name(cluster=w251, "Experiment"="Experiment subVI") -> (w240:refnum<class "Sweep Control.lvclass">)
        n81 = call <userlib>:"Write Experiment Description.vi"("error in (no error)"=w247, "Experiment Description"="Experiment Description", "Control Experiment in"=w256) -> ("error out"=w248:errorcluster, "Control Experiment out"=w255:refnum<class "Control Experiment.lvclass">)  [unwired: 7 in]
        n82 = call <userlib>:"Write Experiment Folder.vi"("error in (no error)"=w248, "Experiment Folder"="Experiment Folder", "Control Experiment in"=w255) -> ("error out"=w249:errorcluster, "Control Experiment out"=w257:refnum<class "Control Experiment.lvclass">)  [unwired: 7 in]
        n83 = call <userlib>:"Read Instruments.vi"("error in (no error)"=w249, "Control Experiment in"=w257) -> ("error out"=w242:errorcluster, "Instruments"=w244:T29, "Control Experiment out"=w243:refnum<class "Control Experiment.lvclass">)  [unwired: 7 in]
        n84 = call <userlib>:"Write Dependencies.vi"("error in (no error)"=w242, "Control Experiment"=w243) -> ("error out"=w238:errorcluster, "Transport out"=w241:refnum<class "Transport.lvclass">)  [unwired: 8 in]
        n85 = call <userlib>:"Write Dependencies.vi"("error in (no error)"=w238, "Transport"=w241, "SweepControl in"=w240) -> ("error out"=w237:errorcluster, "SweepControl out"=w239:refnum<class "Sweep Control.lvclass">)  [unwired: 7 in]
        n86 = Bundle By Name(cluster=w246, "SweepControl"=w239, "Instruments"=w244) -> (w245:T30)
        n87 = call <vilib>:"Add State(s) to Queue__jki_lib_state_machine.vi"("State(s) in (\"\")"=w260) -> ("States Out"=w259:string)  [unwired: 14 in]
      }
      frame "Sweep: Initialize Transport" {
        # "Template Separator\n(You can make a copy of, or modify, this frame)"
        n88 = Unbundle By Name(w270) -> ("SweepControl"=w262:refnum<class "Sweep Control.lvclass">)
        n89 = call <userlib>:"Read Dependencies.vi"("SweepControl in"=w262) -> ("Transport"=w265:refnum<class "Transport.lvclass">, "SweepControl out"=w261:refnum<class "Sweep Control.lvclass">)  [unwired: 8 in, 1 out]
        n90 = Obtain Notifier(notification data type=FALSE, error in (no error)=w269) -> (notifier out=w266:refnum<notifier>, error out=w267:errorcluster)  [unwired: 2 in, 1 out]
        n91 = call <userlib>:"Write notifier.vi"("error in (no error)"=w267, "notifier"=w266, "Transport in"=w265) -> ("error out"=w268:errorcluster, "Transport out"=w264:refnum<class "Transport.lvclass">)  [unwired: 7 in]
        n92 = call <userlib>:"Write Dependencies.vi"("Transport"=w264, "SweepControl in"=w261) -> ("SweepControl out"=w263:refnum<class "Sweep Control.lvclass">)  [unwired: 8 in, 1 out]
        n93 = Bundle By Name(cluster=w270, "SweepControl"=w263, "Notifier"=w266) -> (w271:T30)
        n94 = call <vilib>:"Add State(s) to Queue__jki_lib_state_machine.vi"("State(s) in (\"\")"=w274) -> ("States Out"=w273:string)  [unwired: 14 in]
      }
      frame "Sweep: Prepare JSON" {
        n95 = Unbundle By Name(w295) -> ("SweepControl"=w279:refnum<class "Sweep Control.lvclass">, "B field values"=w277:dbl[], "SweepControl"=w282:refnum<class "Sweep Control.lvclass">, "Instruments.Lockin"=w280:refnum<class "Instrument.Lockin.lvclass">, "Instruments.KH7008"=w289:refnum<class "Inst.Krohn-Hite-7008.lvclass">)
        n96 = call <userlib>:"Read Dependencies.vi"("error in (no error)"=w276, "SweepControl in"=w282) -> ("error out"=w290:errorcluster, "Transport"=w292:refnum<class "Transport.lvclass">)  [unwired: 7 in, 1 out]
        n97 = call <userlib>:"Read Dependencies.vi"("error in (no error)"=w290, "Transport"=w292) -> ("error out"=w291:errorcluster, "C.E."=w293:refnum<class "Control Experiment.lvclass">)  [unwired: 7 in, 1 out]
        n98 = Unbundle By Name(w279) -> ("Experiment"=w278:T6)
        n99 = call <userlib>:"Read Experiment Configuration.vi"("error in (no error)"=w291, "Control Experiment in"=w293) -> ("error out"=w299:errorcluster, "Experiment Description"=w287:T11, "Control Experiment out"=w298:refnum<class "Control Experiment.lvclass">)  [unwired: 7 in]
        n100 = call <userlib>:"Read Wiring Configuration.vi"("error in (no error)"=w299, "Control Experiment in"=w298) -> ("error out"=w281:errorcluster, "Wiring Configuration"=w283:T15)  [unwired: 7 in, 1 out]
        n101 = call <userlib>:"getAO.vi"("error in (no error)"=w276, "Instrument.Lockin in"=w280) -> ("error out"=w300:errorcluster, "AOconfig"=w285:T16, "Instrument.Lockin out"=w301:refnum<class "Instrument.Lockin.lvclass">)  [unwired: 7 in]
        n102 = for {
          N: 1 -> [_]
          tunnel: w289 -> [w307]
          tunnel: [w305] -> w286 mode=concatenating
          tunnel: w276 -> [w304]
          tunnel: [w306] -> w296
          n103 = call-dynamic "getAllChannels.vi"("error in (no error)"=w304, "Inst.Krohn-Hite-7008 in"=w307) -> ("error out"=w306:errorcluster, "allChannelProperties"=w305:T21)  [unwired: 7 in, 1 out]
        }
        n104 = call <userlib>:"getREF.vi"("error in (no error)"=w300, "Instrument.Lockin in"=w301) -> ("error out"=w297:errorcluster, "REFconfig"=w284:T19)  [unwired: 7 in, 1 out]
        n105 = Bundle By Name(cluster=w295, "ContinuousB_JSON.Continuous B Sweep.Experiment"=w278, "ContinuousB_JSON.Continuous B Sweep.B field values"=w277, "ContinuousB_JSON.Experiment Description"=w287, "ContinuousB_JSON.Wiring Configuration"=w283, "ContinuousB_JSON.Lockin.AOconfig"=w285, "ContinuousB_JSON.Lockin.REFconfig"=w284, "ContinuousB_JSON.Krohn Hite.Channel Setting"=w286) -> (w294:T30)
        n106 = Merge Errors(w281, w297, w296) -> (w288:errorcluster)
        n107 = call <vilib>:"Add State(s) to Queue__jki_lib_state_machine.vi"("State(s) in (\"\")"=w303) -> ("States Out"=w302:string)  [unwired: 14 in]
      }
      frame "Sweep: Write JSON" {
        n108 = Unbundle By Name(w329) -> ("SweepControl"=w320:refnum<class "Sweep Control.lvclass">, "ContinuousB_JSON"=w312:T10)
        n109 = call <userlib>:"Read Dependencies.vi"("error in (no error)"=w318, "SweepControl in"=w320) -> ("error out"=w317:errorcluster, "Transport"=w327:refnum<class "Transport.lvclass">, "SweepControl out"=w322:refnum<class "Sweep Control.lvclass">)  [unwired: 7 in]
        n110 = call <userlib>:"Read Dependencies.vi"("error in (no error)"=w317, "Transport"=w327) -> ("error out"=w309:errorcluster, "C.E."=w311:refnum<class "Control Experiment.lvclass">, "Transport"=w323:refnum<class "Transport.lvclass">)  [unwired: 7 in]
        n111 = call <userlib>:"Write JSON to Dictionary.vi"("error in (no error)"=w309, "Control Experiment in"=w311) -> ("error out"=w308:errorcluster, "Control Experiment out"=w310:refnum<class "Control Experiment.lvclass">)  [unwired: 8 in]
        n112 = call "To JSON Text.vim"("error in (no error)"=w308, "Anything"=w312) -> ("error out"=w316:errorcluster, "<JSON>"=w326:string)  [unwired: 8 in]
        n113 = call <userlib>:"Write Dictionary Element.vi"("error in (no error)"=w316, "value"=w326, "key"="<ContinuousB>", "Control Experiment in"=w310) -> ("error out"=w315:errorcluster, "Control Experiment out"=w324:refnum<class "Control Experiment.lvclass">)  [unwired: 6 in]
        n114 = call <userlib>:"Write Dependencies.vi"("error in (no error)"=w315, "Control Experiment"=w324, "Transport in"=w323) -> ("error out"=w314:errorcluster, "Transport out"=w321:refnum<class "Transport.lvclass">)  [unwired: 7 in]
        n115 = call <userlib>:"Write Dependencies.vi"("error in (no error)"=w314, "Transport"=w321, "SweepControl in"=w322) -> ("error out"=w313:errorcluster, "SweepControl out"=w319:refnum<class "Sweep Control.lvclass">)  [unwired: 7 in]
        n116 = Bundle By Name(cluster=w329, "SweepControl"=w319) -> (w328:T30)
        n117 = call <vilib>:"Add State(s) to Queue__jki_lib_state_machine.vi"("State(s) in (\"\")"=w331) -> ("States Out"=w330:string)  [unwired: 14 in]
      }
      frame "Sweep: Simulate Sweep" {
        # "Sweep Rate"
        # "B Field Values"
        # "Template Separator\n(You can make a copy of, or modify, this frame)"
        n118 = Unbundle By Name(w335) -> ("Sweep rate (T/min)"=w334:dbl, "B field values"=w333:dbl[])
        n119 = Array Size(array=w333) -> (size(s)=w336:i32)
        n120 = Decrement(x=w336) -> (x-1=w337:i32)
        n121 = for {
          N: w337 -> [_]
          tunnel: w334 -> [w359]
          tunnel: w333 -> [w367]
          tunnel: [w360] -> w338 mode=indexing
          i -> [w365]
          n122 = Increment(x=w365) -> (x+1=w366:i32)
          n123 = Index Array(array=w367, index #1=w365, index #2=w366) -> (element #1=w363:dbl, element #2=w364:dbl)
          n124 = Subtract(x=w363, y=w364) -> (x-y=w362:dbl)
          n125 = Absolute Value(x=w362) -> (abs(x)=w361:dbl)
          n126 = Divide(x=w361, y=w359) -> (x/y=w360:dbl)
        }
        n127 = for {
          tunnel: w333 -> [w351] mode=indexing
          i -> [w352]
          stop <- w349 stop-if-true
          n128 = local read "B Field Graph"() -> (w355:cluster{i32[], dbl[]}[])
          n129 = Build Array(w352) -> (w357:i32[])
          n130 = Build Array(w351) -> (w356:dbl[])
          n131 = local read "stop"() -> (w349:bool)
          n132 = Bundle(w357, w356) -> (w353:cluster{i32[], dbl[]})  [unwired: 1 in]
          n133 = local write "Setpoint (T)"(w351) -> ()
          n134 = local write "Step #"(w352) -> ()
          n135 = Index Array(array=w355) -> (element=w354:cluster{i32[], dbl[]})  [unwired: 1 in]
          n136 = Build Array(w354, w353) -> (w350:cluster{i32[], dbl[]}[])
          n137 = local write "B Field Graph"(w350) -> ()
          n138 = call <userlib>:"Wait (ms)__ogtk.vi"("milliseconds to wait"=u32 250) -> ()  [unwired: 9 in, 2 out]
        }
        n139 = Get Date/Time In Seconds() -> (seconds since 1Jan1904=w341:timestamp)
        n140 = Add Array Elements(numeric array=w338) -> (sum=w343:dbl)
        n141 = Quotient & Remainder(x=w343, y=60.0) -> (x-y*floor(x/y)=→"time (minutes)":dbl, floor(x/y)=→"time (hours)":dbl)
        n142 = Multiply(x=w343, y=60.0) -> (x*y=w340:dbl)
        n143 = Add(x=w340, y=w341) -> (x+y=→"ETA":timestamp)
        n144 = call <vilib>:"Add State(s) to Queue__jki_lib_state_machine.vi"("State(s) in (\"\")"=w348) -> ("States Out"=w347:string)  [unwired: 14 in]
      }
      frame "Sweep: Sweep" {
        n145 = Unbundle By Name(w372) -> ("Instruments.Magnet"=w381:refnum<class "Instrument.Cryostat.lvclass">, "B field values"=w368:dbl[], "Sweep rate (T/min)"=w382:dbl, "Notifier"=w383:refnum<notifier>, "SweepControl"=w369:refnum<class "Sweep Control.lvclass">)
        n146 = Bundle By Name(cluster=w369, "Lockin_Sweep Configuration"="Lockin_sweep Configuration") -> (w379:refnum<class "Sweep Control.lvclass">)
        n147 = while {
          tunnel: w383 -> [w415]
          tunnel: w380 -> [w404]
          tunnel: [w417] -> w385
          tunnel: [w416] -> w378
          shift-right: [w413] -> _
          shift-left: 0 -> [w410]
          tunnel: w368 -> [w398]
          tunnel: w382 -> [w396]
          tunnel: "Mode" -> [w400]
          shift-right: [w399] -> w370
          shift-left: w381 -> [w403]
          i -> [w409]
          stop <- w407 stop-if-true
          # "setpoint"
          # "ramp rate"
          # "Loop that sends notifications"
          n148 = Array Size(array=w398) -> (size(s)=w408:i32)
          n149 = Decrement(x=w408) -> (x-1=w411:i32)
          n150 = Index Array(array=w398, index=w410) -> (element=w397:dbl)
          "Setpoint (T)" <- w397
          n151 = Greater Or Equal?(x=w409, y=w411) -> (x >= y?=w412:bool)
          n152 = Or(x="stop", y=w412) -> (x .or. y?=w414:bool)
          n153 = Or(x=w414, y=w404) -> (x .or. y?=w407:bool)
          n154 = call-dynamic "Set Magnet.vi"("Mode"=w400, "error in (no error)"=w404, "Target Rate (T/min)"=w396, "Target Field (T)"=w397, "Instrument.Cryostat in"=w403) -> ("error out"=w401:errorcluster, "Instrument.Cryostat out"=w402:refnum<class "Instrument.Cryostat.lvclass">)  [unwired: 5 in]
          n155 = call <userlib>:"Wait for Magnet Setpoint.vi"("error in (no error)"=w401, "Setpoint (T)"=w397, "Instrument.Cryostat in"=w402) -> ("error out"=w406:errorcluster, "Instrument.Cryostat out"=w399:refnum<class "Instrument.Cryostat.lvclass">)  [unwired: 7 in]
          n156 = Send Notification(notification=w407, notifier=w415, error in (no error)=w406) -> (notifier out=w417:refnum<notifier>, error out=w416:errorcluster)
          n157 = Increment(x=w410) -> (x+1=w413:i32)
          "Step #" <- w409
        }
        n158 = while {
          tunnel: w380 -> [w390]
          tunnel: w383 -> [w391]
          tunnel: [w392] -> w376
          tunnel: w379 -> [w389]
          stop <- w395 stop-if-true
          # "Loop that listens to notifications"
          n159 = call "Take Measurement.vi"("error in (no error)"=w390, "SweepControl in"=w389) -> ("error out"=w388:errorcluster)  [unwired: 8 in, 1 out]
          n160 = Get Notifier Status(notifier=w391, error in (no error)=w388) -> (current notification=w394:bool, error out=w393:errorcluster)  [unwired: 3 out]
          n161 = Or(x=w394, y=w393) -> (x .or. y?=w395:bool)
          n162 = call <vilib>:"Clear Errors.vi"("error in (no error)"=w393) -> ("error out"=w392:errorcluster)  [unwired: 5 in, 1 out]
        }
        n163 = Bundle By Name(cluster=w372, "Instruments.Magnet"=w370) -> (w371:T30)
        n164 = Merge Errors(w378, w376) -> (w375:errorcluster)
        n165 = Release Notifier(notifier=w385, error in (no error)=w375) -> (error out=w377:errorcluster)  [unwired: 1 in, 2 out]
        n166 = call <vilib>:"Add State(s) to Queue__jki_lib_state_machine.vi"("State(s) in (\"\")"=w387) -> ("States Out"=w386:string)  [unwired: 14 in]
      }
    }
  }
  "error out" <- w1
